vi "Send Arm Trigger.vi"(8 "error in (no error)":errorcluster, 11 "VISA resource name":refnum<visa-resource-name>) -> (0 "error out":errorcluster, 3 "VISA resource name out":refnum<visa-resource-name>)   [LabVIEW 2014, in "Fluke 190 Series II.lvlib"]
doc: "Resets and arms the trigger system for a new acquisition. It can also be used for single shot acquisitions. When it is given while an acquisition is in progress, this acquisition is aborted and the trigger system is rearmed. It can also be used to go from other modes (e.g. from Replay mode) to 'live' acquisition mode."
uses:
  Fluke 190 Series II.lvlib
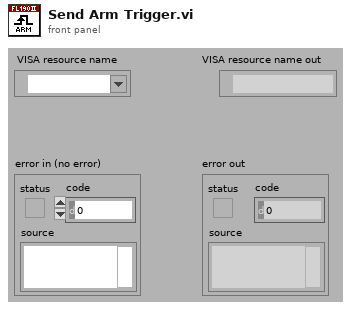
[diagram p1: front panel]
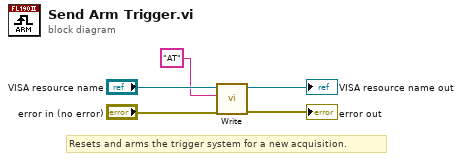
[diagram p0: block diagram]
diagram:
  # "Resets and arms the trigger system for a new acquisition."
  n1 = call "Write.vi"("error in (no error)"="error in (no error)", "Write Buffer"="AT", "VISA resource name"="VISA resource name") -> ("error out"=→"error out":errorcluster, "VISA resource name out"=→"VISA resource name out":refnum<visa-resource-name>)  [unwired: 7 out]
